vi "setConfiguration.vi"(8 "error in (no error)":errorcluster, 10 "configuration":cluster{"intensities":u32[], "on_states":u8[]}, 11 "Xcite in":refnum<class "Xcite.lvclass">) -> (0 "error out":errorcluster, 3 "Xcite out":refnum<class "Xcite.lvclass">)   [LabVIEW 2019, in "Xcite.lvclass"]
doc: "Sets the inensity and on/off state of each channel in the XCite device."
uses:
  Xcite.lvclass
  Xcite.lvclass/Xcite.ctl
  etc.xcite/XCite.lvlib
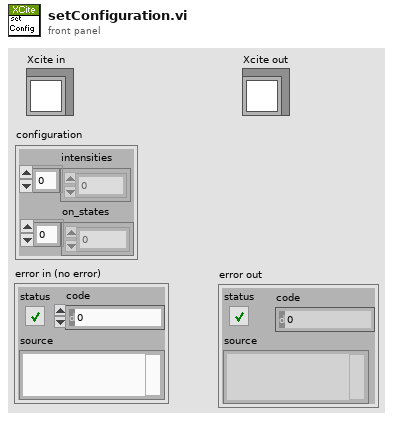
[diagram p1: front panel]
types:
  T1 = cluster{"serial":u32, "type":u16, "name":string, "wavelenghts_vec":u32[], "exclusivity_vec":u32[], "intensity_max_vec":u32[], "intensity_min_vec":u32[]}
  T2 = cluster{"LightSourceName":string, "hDevice":u64, "hCamera":u64, "iNumChannels":i32, "iNumWheels":i32, "dwSystemState":u32, "dwSerialNumber":u32, "dwSystemCaps":u32, "iLastChannelOnWheel":i16[], "XCiteChannels":cluster{"szLedName":string, "iWaveLength":i32, "IBelongToWheelNumber":i32, "iIntensity":i32, "iIntensityMin":i32, "iIntensityMax":i32, "iIntensityStep":i32, "iExtTriggerNum":i32, "iLedTemp":i32, "dwLEDState":u32}[]}
  T3 = cluster{"szLedName":string, "iWaveLength":i32, "IBelongToWheelNumber":i32, "iIntensity":i32, "iIntensityMin":i32, "iIntensityMax":i32, "iIntensityStep":i32, "iExtTriggerNum":i32, "iLedTemp":i32, "dwLEDState":u32}[]
  T4 = cluster{"szLedName":string, "iWaveLength":i32, "IBelongToWheelNumber":i32, "iIntensity":i32, "iIntensityMin":i32, "iIntensityMax":i32, "iIntensityStep":i32, "iExtTriggerNum":i32, "iLedTemp":i32, "dwLEDState":u32}
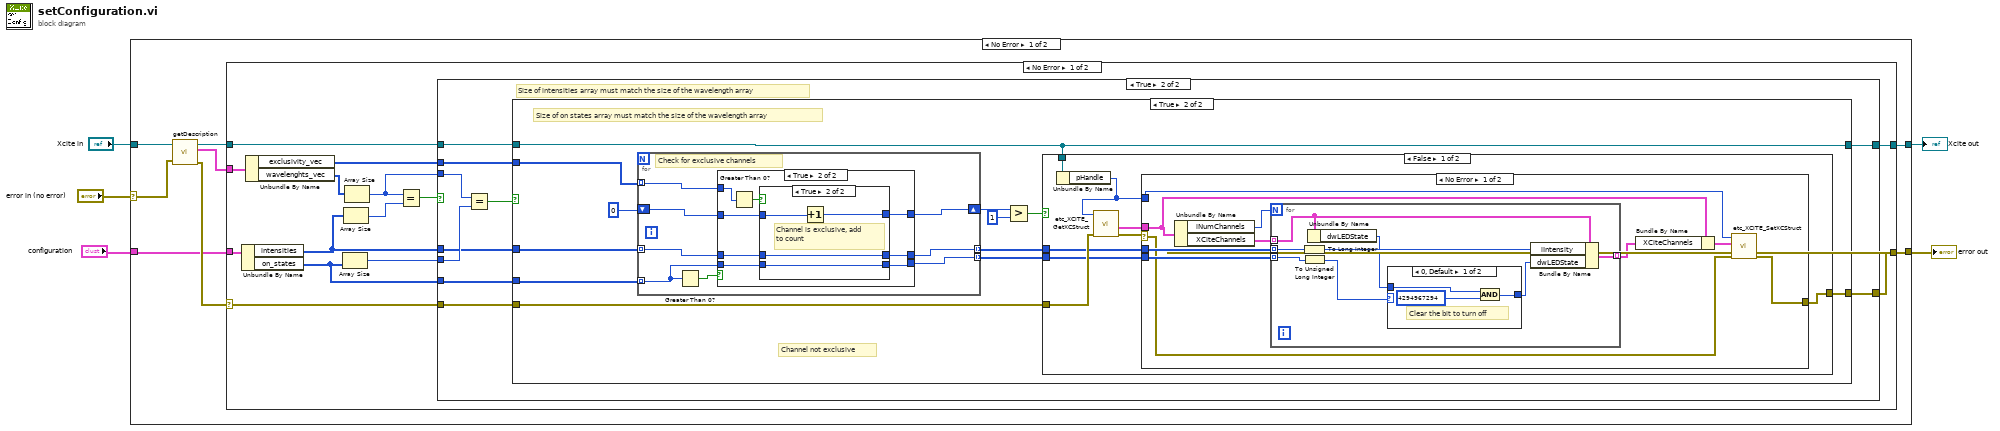
[diagram p0: block diagram]
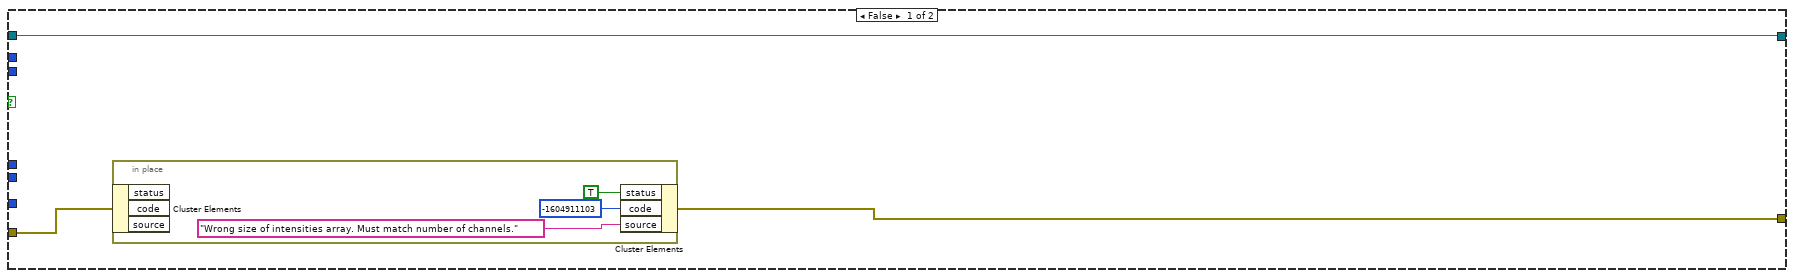
[diagram p2: hidden frame]
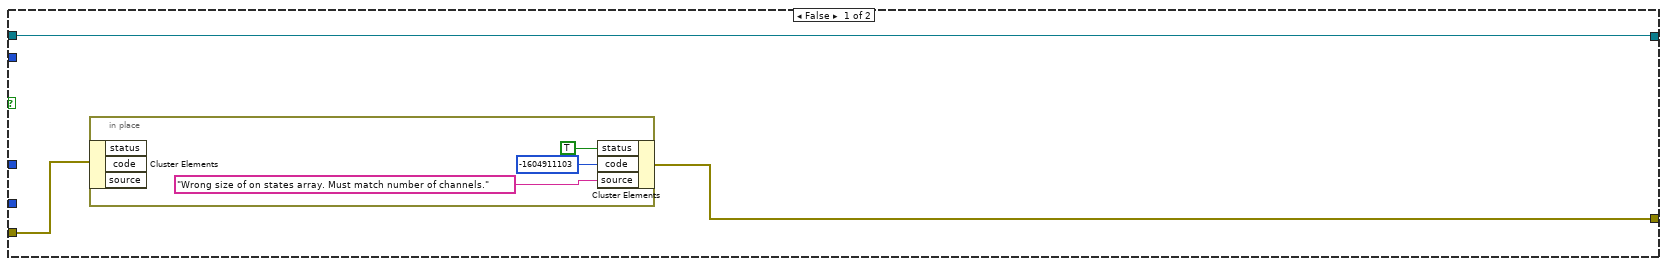
[diagram p3: hidden frame]
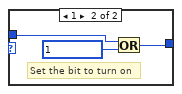
[diagram p4: hidden frame]
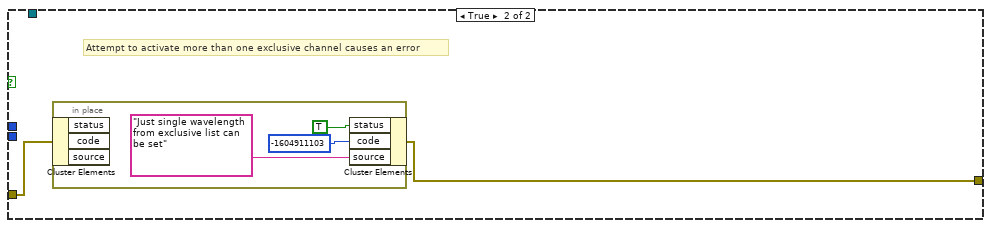
[diagram p6: hidden frame]
diagram:
  n1 = case shown="No Error" "error in (no error)" {
    selector: "error in (no error)" -> [w8 w129]
    tunnel: [w13 w129] -> w4
    tunnel: "Xcite in" -> [w11 w128]
    tunnel: [w12 w128] -> w2
    tunnel: "configuration" -> [w6 _]
    frame No Error {
      n2 = call "getDescription.vi"("error in (no error)"=w8, "Xcite in"=w11) -> ("error out"=w9:errorcluster, "description"=w7:T1, "Xcite out"=w10:refnum<class "Xcite.lvclass">)  [unwired: 7 in]
      n3 = case shown="No Error" w9 {
        selector: w9 -> [w24 w126]
        tunnel: [w27 w126] -> w13
        tunnel: [w26 w127] -> w12
        tunnel: w10 -> [w25 w127]
        tunnel: w7 -> [w23 _]
        tunnel: w6 -> [w21 _]
        frame No Error {
          n4 = Unbundle By Name(w21) -> ("intensities"=w15:u32[], "on_states"=w14:u8[])
          n5 = Unbundle By Name(w23) -> ("exclusivity_vec"=w16:u32[], "wavelenghts_vec"=w22:u32[])
          n6 = Array Size(array=w14) -> (size(s)=w18:i32)
          n7 = Array Size(array=w15) -> (size(s)=w20:i32)
          n8 = Array Size(array=w22) -> (size(s)=w17:i32)
          n9 = Equal?(x=w17, y=w20) -> (x = y?=w19:bool)
          n10 = case shown="True" w19 {
            tunnel: [w29 w43] -> w27
            tunnel: [w28 w42] -> w26
            tunnel: w25 -> [w28 w41]
            tunnel: w24 -> [w30 w40]
            tunnel: w18 -> [_ w38]
            tunnel: w17 -> [_ w39]
            tunnel: w16 -> [_ w36]
            tunnel: w15 -> [_ w35]
            tunnel: w14 -> [_ w34]
            frame False {
              n11 = in-place {
                n12 = in-place-cluster #1(w30) -> ()  [unwired: 3 out]
                n13 = in-place-cluster #1("status"=TRUE, "code"=-1604911103, "source"="Wrong size of intensities array. Must match number of channels.") -> (w29:errorcluster)
              }
            }
            frame True {
              # "Size of intensities array must match the size of the wavelength array"
              n14 = Equal?(x=w39, y=w38) -> (x = y?=w37:bool)
              n15 = case shown="True" w37 {
                tunnel: [w45 w51] -> w43
                tunnel: [w44 w50] -> w42
                tunnel: w41 -> [w44 w50]
                tunnel: w40 -> [w46 w52]
                tunnel: w36 -> [_ w59]
                tunnel: w35 -> [_ w61]
                tunnel: w34 -> [_ w60]
                frame False {
                  n16 = in-place {
                    n17 = in-place-cluster #2(w46) -> ()  [unwired: 3 out]
                    n18 = in-place-cluster #2("status"=TRUE, "code"=-1604911103, "source"="Wrong size of on states array. Must match number of channels.") -> (w45:errorcluster)
                  }
                }
                frame True {
                  # "Channel not exclusive"
                  # "Size of on states array must match the size of the wavelength array"
                  n19 = for {
                    tunnel: w61 -> [w106] mode=indexing
                    tunnel: w60 -> [w105] mode=indexing
                    tunnel: w59 -> [w104] mode=indexing
                    shift-right: [w102] -> w57
                    shift-left: u16 0 -> [w103]
                    tunnel: [w101] -> w54 mode=indexing
                    tunnel: [w100] -> w53 mode=indexing
                    # "Check for exclusive channels"
                    n20 = Greater Than 0?(x=w105) -> (x > 0?=w107:bool)
                    n21 = case shown="True" w107 {
                      tunnel: w106 -> [w109 w115]
                      tunnel: w105 -> [w110 w113]
                      tunnel: w104 -> [_ w118]
                      tunnel: [w110 w112] -> w100
                      tunnel: [w109 w114] -> w101
                      tunnel: w103 -> [w108 w116]
                      tunnel: [w108 w111] -> w102
                      frame False {
                      }
                      frame True {
                        n22 = Greater Than 0?(x=w118) -> (x > 0?=w117:bool)
                        n23 = case shown="True" w117 {
                          tunnel: w116 -> [w121 w125]
                          tunnel: [w121 w124] -> w111
                          tunnel: w115 -> [w120 w123]
                          tunnel: [w120 w123] -> w114
                          tunnel: w113 -> [w119 w122]
                          tunnel: [w119 w122] -> w112
                          frame False {
                            # "Channel not exclusive"
                          }
                          frame True {
                            # "Channel is exclusive, add to count"
                            n24 = Increment(x=w125) -> (x+1=w124:u16)
                          }
                        }
                      }
                    }
                  }
                  n25 = Greater?(x=w57, y=u16 1) -> (0:w55:bool)
                  n26 = case shown="False" w55 {
                    tunnel: w54 -> [w66 _]
                    tunnel: w53 -> [w65 _]
                    tunnel: w52 -> [w69 w96]
                    tunnel: [w63 w95] -> w51
                    tunnel: w50 -> [w67 _]
                    frame False {
                      n27 = Unbundle By Name(w67) -> ("pHandle"=w62:u64)
                      n28 = call "etc_XCITE_GetXCStruct.vi"("error in (no error)"=w69, "h"=w62) -> ("error out"=w68:errorcluster, "XCiteStructure"=w64:T2)  [unwired: 6 in, 2 out]
                      n29 = case shown="No Error" w68 {
                        selector: w68 -> [w75 w94]
                        tunnel: w66 -> [w77 _]
                        tunnel: w65 -> [w76 _]
                        tunnel: w64 -> [w72 _]
                        tunnel: [w74 w94] -> w63
                        tunnel: w62 -> [w73 _]
                        frame No Error {
                          n30 = Unbundle By Name(w72) -> ("iNumChannels"=w79:i32, "XCiteChannels"=w78:T3)
                          n31 = for {
                            N: w79 -> [_]
                            tunnel: w78 -> [w84] mode=indexing
                            tunnel: w77 -> [w87] mode=indexing
                            tunnel: w76 -> [w86] mode=indexing
                            tunnel: [w80] -> w71 mode=indexing
                            n32 = To Long Integer(number=w87) -> (32bit integer=w85:i32)
                            n33 = To Unsigned Long Integer(number=w86) -> (unsigned 32bit integer=w83:u32)
                            n34 = Unbundle By Name(w84) -> ("dwLEDState"=w82:u32)
                            n35 = case shown="0, Default" w83 {
                              tunnel: w82 -> [w90 w93]
                              tunnel: [w88 w91] -> w81
                              frame 0, Default {
                                # "Clear the bit to turn off"
                                n36 = And(x=w90, y=u32 4294967294) -> (x .and. y?=w88:u32)
                              }
                              frame 1 {
                                # "Set the bit to turn on"
                                n37 = Or(x=w93, y=u32 1) -> (x .or. y?=w91:u32)
                              }
                            }
                            n38 = Bundle By Name(cluster=w84, "iIntensity"=w85, "dwLEDState"=w81) -> (w80:T4)
                          }
                          n39 = Bundle By Name(cluster=w72, "XCiteChannels"=w71) -> (w70:T2)
                          n40 = call "etc_XCITE_SetXCStruct.vi"("error in (no error)"=w75, "XCiteStructure"=w70, "h"=w73) -> ("error out"=w74:errorcluster)  [unwired: 6 in, 2 out]
                        }
                        frame Error {
                        }
                      }
                    }
                    frame True {
                      # "Attempt to activate more than one exclusive channel causes an error"
                      n41 = in-place {
                        n42 = in-place-cluster #3(w96) -> ()  [unwired: 3 out]
                        n43 = in-place-cluster #3("status"=TRUE, "code"=-1604911103, "source"="Just single wavelength from exclusive list can be set") -> (w95:errorcluster)
                      }
                    }
                  }
                }
              }
            }
          }
        }
        frame Error {
        }
      }
    }
    frame Error {
    }
  }
  "Xcite out" <- w2
  "error out" <- w4
